vi "modbus slave全局.vi"() -> ()   [LabVIEW 2016]
panel:
  in  "与CODMn交互全局":T1 {"加标回收启动时间" format="%<%Y/%m/%d %H:%M:%S>T"; "水样启动时间" format="%<%Y/%m/%d %H:%M:%S>T"}
  in  "执行结果反馈":u16[](array[numeric])
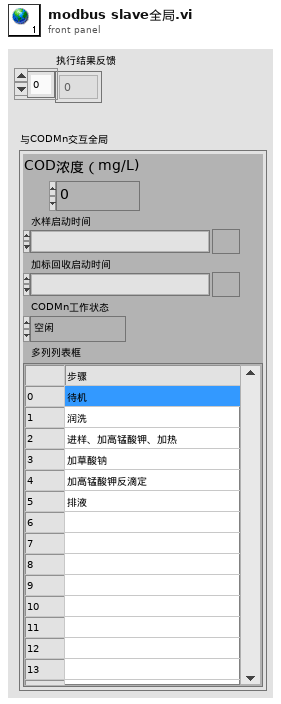
[diagram p1: front panel]
types:
  T1 = cluster{"COD浓度（mg/L)":dbl, "水样启动时间":timestamp, "加标回收启动时间":timestamp, "CODMn工作状态":enum16{"空闲", "水样测试", "标样核查", "零点核查", "跨度核查", "空白测试", "平行样测试", "加标回收", "空白校准", "标样校准", "初始化（清洗）"}, "多列列表框":i32}
diagram:
